vi "Scale.vi"(1 "B_start":dbl, 2 "B_latest":dbl, 3 "Total_curves":i32) -> (0 "output cluster":cluster{"Offset":dbl, "Multiplier":dbl})   [LabVIEW 2016]
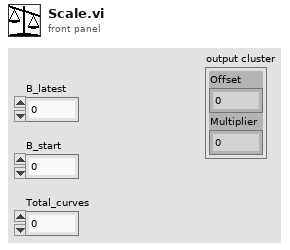
[diagram p1: front panel]
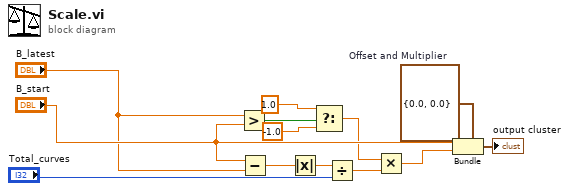
[diagram p0: block diagram]
diagram:
  w2 = cluster{"Offset":dbl, "Multiplier":dbl} {"Offset"=0.0, "Multiplier"=0.0}  # Offset and Multiplier
  n1 = Greater?(x="B_latest", y="B_start") -> (0:w4:bool)
  n2 = Subtract(x="B_start", y="B_latest") -> (x-y=w3:dbl)
  n3 = Absolute Value(x=w3) -> (abs(x)=w9:dbl)
  n4 = Select(t=1.0, s=w4, f=-1.0) -> (s? t:f=w7:dbl)
  n5 = Divide(x=w9, y="Total_curves") -> (x/y=w11:dbl)
  n6 = Multiply(x=w7, y=w11) -> (x*y=w8:dbl)
  n7 = Bundle(cluster=w2, "Offset"="B_start", "Multiplier"=w8) -> (→"output cluster":cluster{"Offset":dbl, "Multiplier":dbl})
